vi "HEWH Extract Draw Data.vi"(5 "Test Type":T1, 8 "error in (no error)":errorcluster, 11 "UEF Calculated Values in":T2 {"Data Indexes"."15 sec after Draw Index" format="%#.2f"; "Data Indexes"."15 sec after Draw Timestamp" format="%#.2f"; "Data Indexes"."Test Start Timestamp" format="%.2f"; "Data Indexes"."Test End Timestamp" format="%.2f"; "Data Indexes"."T0 Timestamp" format="%.2f"; "Data Indexes"."Tsf Timestamp" format="%.2f"; "Data Indexes"."Tsu0 Timestamp" format="%.2f"; "Data Indexes"."Tmax1 Timestamp" format="%.2f"; "Data Indexes"."Draw Index Timestamp" format="%#.2f"; "Data Indexes"."Non-Draw Timestamp" format="%#.2f"; "Data Indexes"."Heating Timestamp" format="%#.2f"; "Data Indexes"."Start Energy (BTU-Gas)" format="%.6f"; "Data Indexes"."Start Watt Hours" format="%.6f"; "Static Data"."V - Volume of Wh (True)" format="%.5f"; "Static Data"."T-Ambinet Nominal (°F)" format="%.5f"; "Static Data"."T-Inlet Setpoint (°F)" format="%.5f"; "Static Data"."T-Wh Setpoint (°F)" format="%.5f"; "Sampled Data"."Qe (Wh)" format="%.5f"; "Sampled Data"."Tau stby2 (hr)" format="%.5f"; "Sampled Data"."Tastby2 (°F)" format="%.5f"; "Sampled Data"."Qf (BTU)" format="%.5f"; "Sampled Data"."Qe (BTU)" format="%.5f"; "Sampled Data"."Tmax1 (°F)" format="%.5f"; "Sampled Data"."T0 (°F)" format="%.5f"; "Sampled Data"."Qr (BTU)" format="%.5f"; "Sampled Data"."T 24(°F)" format="%.5f"; "Sampled Data"."T astby(°F)" format="%.5f"; "Sampled Data"."T tstby(°F)" format="%.5f"; "Sampled Data"."T su0(°F)" format="%.5f"; "Sampled Data"."T suf(°F)" format="%.5f"; "Sampled Data"."Tau stby_1 (hr)" format="%.5f"; "Sampled Data"."Qsuf (BTU)" format="%.5f"; "Sampled Data"."Qsu0 (BTU)" format="%.5f"; "Calculated Values"."Draw Bonus Volume (gal)" format="%.6f"; "Calculated Values"."Adjustment Factor" format="%.6f"; "Calculated Values"."T*avg_del(n-1)" format="%.6f"; "Calculated Values"."T*min(n-1)" format="%.6f"; "Calculated Values"."T*avg_del(n)" format="%.6f"; "Calculated Values"."Vn" format="%.6f"; "Calculated Values"."Qdm (BTU)" format="%.6f"; "Calculated Values"."QHWD (BTU)" format="%.6f"; "Calculated Values"."QHW (BTU)" format="%.6f"; "Calculated Values"."UEF" format="%.6f"; "Calculated Values"."QHW67 (BTU)" format="%.6f"; "Calculated Values"."Qda (BTU)" format="%.6f"; "Calculated Values"."Qd (BTU)" format="%.6f"; "Calculated Values"."Q (BTU)" format="%.6f"; "Calculated Values"."UA (BTU/(hr*F))" format="%.6f"; "Calculated Values"."Qhr (BTU/hr)" format="%.6f"; "Calculated Values"."Qstby (BTU)" format="%.6f"; "Calculated Values"."nu_r" format="%.6f"; "Calculated Values"."CpUEF (BTU/(lb*F))" format="%.6f"; "Calculated Values"."rho_nu (lb/gal)" format="%.6f"; "Calculated Values"."V1- Vol (Gal)" format="%.6f"; "Calculated Values"."M cluster mass removed (lb)" format="%.6f"; "Calculated Values"."Cp theoretical (BTU/(lbm °F))" format="%.6f"; "Calculated Values"."Tin1 - Mean Inlet 1st Cluster (°F)" format="%.6f"; "Calculated Values"."Tdel1-Mean Outlet 1st Cluster(°F)" format="%.6f"; "Calculated Values"."Cp 24 (BTU/(lb*F))" format="%.6f"; "Calculated Values"."Cp standby (BTU/(lb*F))" format="%.6f"; "Calculated Values"."Cp2 (BTU/(lb*F))" format="%.6f"; "Calculated Values"."Cp1 (BTU/(lb*F))" format="%.6f"; "Calculated Values"."rho 24 (lb/gal)" format="%.6f"; "Calculated Values"."rho standby (lb/gal)" format="%.6f"; "Calculated Values"."rho 2 (lb/gal)" format="%.6f"; "Calculated Values"."Density of cold water All (lbm/gal)" format="%#.3g"; "Calculated Values"."CpHW (BTU/(lbm °F))" format="%#.3g"; "Calculated Values"."Density of hot water All (lbm/gal)" format="%#.3g"; "Calculated Values"."Mass of water All (lbm)" format="%#.3f"}) -> (0 "error out":errorcluster, 3 "UEF Calculated Values Out":T2 {"Data Indexes"."15 sec after Draw Index" format="%#.2f"; "Data Indexes"."15 sec after Draw Timestamp" format="%#.2f"; "Data Indexes"."Test Start Timestamp" format="%.2f"; "Data Indexes"."Test End Timestamp" format="%.2f"; "Data Indexes"."T0 Timestamp" format="%.2f"; "Data Indexes"."Tsf Timestamp" format="%.2f"; "Data Indexes"."Tsu0 Timestamp" format="%.2f"; "Data Indexes"."Tmax1 Timestamp" format="%.2f"; "Data Indexes"."Draw Index Timestamp" format="%#.2f"; "Data Indexes"."Non-Draw Timestamp" format="%#.2f"; "Data Indexes"."Heating Timestamp" format="%#.2f"; "Data Indexes"."Start Energy (BTU-Gas)" format="%.6f"; "Data Indexes"."Start Watt Hours" format="%.6f"; "Static Data"."V - Volume of Wh (True)" format="%.5f"; "Static Data"."T-Ambinet Nominal (°F)" format="%.5f"; "Static Data"."T-Inlet Setpoint (°F)" format="%.5f"; "Static Data"."T-Wh Setpoint (°F)" format="%.5f"; "Sampled Data"."Qe (Wh)" format="%.5f"; "Sampled Data"."Tau stby2 (hr)" format="%.5f"; "Sampled Data"."Tastby2 (°F)" format="%.5f"; "Sampled Data"."Qf (BTU)" format="%.5f"; "Sampled Data"."Qe (BTU)" format="%.5f"; "Sampled Data"."Tmax1 (°F)" format="%.5f"; "Sampled Data"."T0 (°F)" format="%.5f"; "Sampled Data"."Qr (BTU)" format="%.5f"; "Sampled Data"."T 24(°F)" format="%.5f"; "Sampled Data"."T astby(°F)" format="%.5f"; "Sampled Data"."T tstby(°F)" format="%.5f"; "Sampled Data"."T su0(°F)" format="%.5f"; "Sampled Data"."T suf(°F)" format="%.5f"; "Sampled Data"."Tau stby_1 (hr)" format="%.5f"; "Sampled Data"."Qsuf (BTU)" format="%.5f"; "Sampled Data"."Qsu0 (BTU)" format="%.5f"; "Calculated Values"."Draw Bonus Volume (gal)" format="%.6f"; "Calculated Values"."Adjustment Factor" format="%.6f"; "Calculated Values"."T*avg_del(n-1)" format="%.6f"; "Calculated Values"."T*min(n-1)" format="%.6f"; "Calculated Values"."T*avg_del(n)" format="%.6f"; "Calculated Values"."Vn" format="%.6f"; "Calculated Values"."Qdm (BTU)" format="%.6f"; "Calculated Values"."QHWD (BTU)" format="%.6f"; "Calculated Values"."QHW (BTU)" format="%.6f"; "Calculated Values"."UEF" format="%.6f"; "Calculated Values"."QHW67 (BTU)" format="%.6f"; "Calculated Values"."Qda (BTU)" format="%.6f"; "Calculated Values"."Qd (BTU)" format="%.6f"; "Calculated Values"."Q (BTU)" format="%.6f"; "Calculated Values"."UA (BTU/(hr*F))" format="%.6f"; "Calculated Values"."Qhr (BTU/hr)" format="%.6f"; "Calculated Values"."Qstby (BTU)" format="%.6f"; "Calculated Values"."nu_r" format="%.6f"; "Calculated Values"."CpUEF (BTU/(lb*F))" format="%.6f"; "Calculated Values"."rho_nu (lb/gal)" format="%.6f"; "Calculated Values"."V1- Vol (Gal)" format="%.6f"; "Calculated Values"."M cluster mass removed (lb)" format="%.6f"; "Calculated Values"."Cp theoretical (BTU/(lbm °F))" format="%.6f"; "Calculated Values"."Tin1 - Mean Inlet 1st Cluster (°F)" format="%.6f"; "Calculated Values"."Tdel1-Mean Outlet 1st Cluster(°F)" format="%.6f"; "Calculated Values"."Cp 24 (BTU/(lb*F))" format="%.6f"; "Calculated Values"."Cp standby (BTU/(lb*F))" format="%.6f"; "Calculated Values"."Cp2 (BTU/(lb*F))" format="%.6f"; "Calculated Values"."Cp1 (BTU/(lb*F))" format="%.6f"; "Calculated Values"."rho 24 (lb/gal)" format="%.6f"; "Calculated Values"."rho standby (lb/gal)" format="%.6f"; "Calculated Values"."rho 2 (lb/gal)" format="%.6f"; "Calculated Values"."Density of cold water All (lbm/gal)" format="%#.3g"; "Calculated Values"."CpHW (BTU/(lbm °F))" format="%#.3g"; "Calculated Values"."Density of hot water All (lbm/gal)" format="%#.3g"; "Calculated Values"."Mass of water All (lbm)" format="%#.3f"})   [LabVIEW 2023]
uses:
  Type Definitions/UEF Constants.ctl
  Type Definitions/HEWH Draw Stats.ctl
  Type Definitions/HEWH FHR Draw Type.ctl
  Type Definitions/FHR Bins.ctl
  Type Definitions/HEWH Meter Type.ctl
  Type Definitions/HEWH Test Type.ctl
  Type Definitions/HEWH Remove 15 Seconds.ctl
  <vilib>/Analysis/baseanly.llb/Mean (DBL).vi
  <vilib>/Analysis/NI_AALBase.lvlib
panel:
  # "FHR"
  # "FHR"
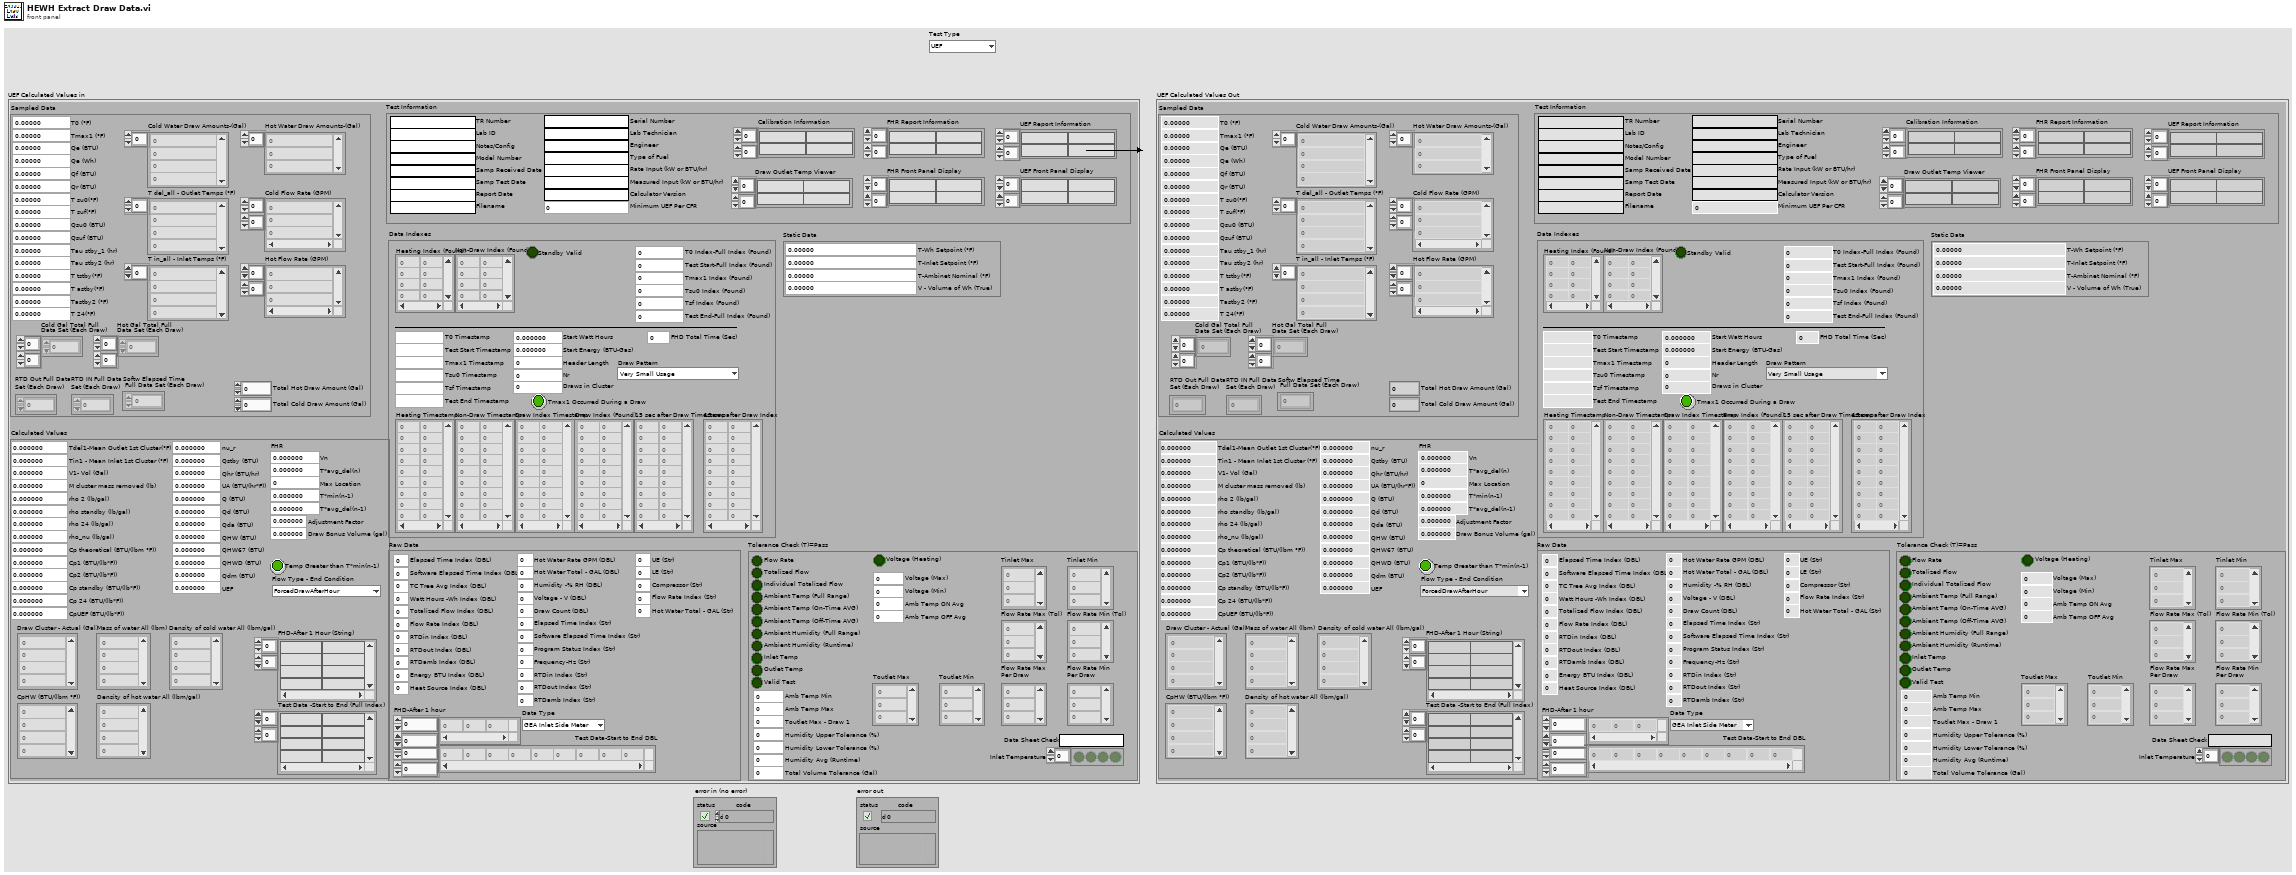
[diagram p1: front panel]
types:
  T1 = typedef "HEWH Test Type.ctl" = enum16{"UEF", "FHD"}
  T2 = typedef "UEF Constants.ctl" = cluster{"Calculated Values":T3, "Sampled Data":cluster{"Cold Water Draw Amounts-(Gal)":dbl[], "T del_all - Outlet Temps (°F)":dbl[], "T in_all - Inlet Temps (°F)":dbl[], "Qsu0 (BTU)":dbl, "Qsuf (BTU)":dbl, "Tau stby_1 (hr)":dbl, "T suf(°F)":dbl, "T su0(°F)":dbl, "T tstby(°F)":dbl, "T astby(°F)":dbl, "T 24(°F)":dbl, "Qr (BTU)":dbl, "T0 (°F)":dbl, "Tmax1 (°F)":dbl, "Qe (BTU)":dbl, "Qf (BTU)":dbl, "Tastby2 (°F)":dbl, "RTD Out Full Data\nSet (Each Draw)":dbl[][], "RTD IN Full Data\nSet (Each Draw)":dbl[][], "Tau stby2 (hr)":dbl, "Hot Water Draw Amounts-(Gal)":dbl[], "Cold Flow Rate (GPM)":dbl[][], "Hot Flow Rate (GPM)":dbl[][], "Softw Elapsed Time\n Full Data Set (Each Draw)":dbl[][], "Cold Gal Total Full\nData Set (Each Draw)":dbl[][], "Total Hot Draw Amount (Gal) ":dbl, "Total Cold Draw Amount (Gal)":dbl, "Qe (Wh)":dbl, "Hot Gal Total Full\nData Set (Each Draw)":dbl[][]}, "Static Data":cluster{"T-Wh Setpoint (°F)":dbl, "T-Inlet Setpoint (°F)":dbl, "T-Ambinet Nominal (°F)":dbl, "V - Volume of Wh (True)":dbl}, "Data Indexes":cluster{"Test Start-Full Index (Found)":i32, "Header Length":i32, "Draw Index (Found)":i32[][], "Nr":i32, "Start Watt Hours":dbl, "Tsu0 Index (Found)":i32, "Tsf Index (Found)":i32, "Start Energy (BTU-Gas)":dbl, "Draws in Cluster":i32, "T0 Index-Full Index (Found)":i32, "Non-Draw Index (Found)":i32[][], "Tmax1 Index (Found)":i32, "Test End-Full Index (Found)":i32, "Heating Index (Found)":i32[][], "Heating Timestamp":dbl[][], "Non-Draw Timestamp":dbl[][], "Draw Index Timestamp":dbl[][], "Tmax1 Timestamp":dbl, "Tsu0 Timestamp":dbl, "Tsf Timestamp":dbl, "T0 Timestamp":dbl, "Test End Timestamp":dbl, "Test Start Timestamp":dbl, "15 sec after Draw Timestamp":dbl[][], "15 sec after Draw Index":dbl[][], "Tmax1 Occurred During a Draw":bool, "FHD Total Time (Sec)":dbl, "Draw Pattern":T5, "Standby Valid":bool}, "Raw Data":cluster{"Elapsed Time Index (DBL)":i32, "Software Elapsed Time Index (DBL)":i32, "TC Tree Avg Index (DBL)":i32, "Watt Hours -Wh Index (DBL)":i32, "Energy BTU Index (DBL)":i32, "Totalized Flow Index (DBL)":i32, "Flow Rate Index (DBL)":i32, "Program Status Index (Str)":i32, "RTDin Index (DBL)":i32, "RTDout Index (DBL)":i32, "RTDamb Index (DBL)":i32, "Test Data-Start to End DBL":dbl[][], "Data Type":T6, "Heat Source Index (DBL)":i32, "Hot Water Rate GPM (DBL)":i32, "Hot Water Total - GAL (DBL)":i32, "FHD-After 1 hour":dbl[][], "Humidity -% RH (DBL)":i32, "Voltage - V (DBL)":i32, "Draw Count (DBL)":i32, "Elapsed Time Index (Str)":i32, "Software Elapsed Time Index (Str)":i32, "Frequency-Hz (Str)":i32, "RTDin Index (Str)":i32, "RTDout Index (Str)":i32, "RTDamb Index (Str)":i32, "UE (Str)":i32, "LE (Str)":i32, "Compressor (Str)":i32, "Flow Rate Index (Str)":i32, "Hot Water Total - GAL (Str)":i32}, "Tolerance Check (T)=Pass":cluster{"Flow Rate":bool, "Totalized Flow":bool, "Ambient Temp (Full Range)":bool, "Ambient Humidity (Full Range)":bool, "Inlet Temp":bool, "Outlet Temp":bool, "Valid Test":bool, "Individual Totalized Flow":bool, "Data Sheet Check":string, "Inlet Temperature":bool[], "Tinlet Max":dbl[], "Tinlet Min":dbl[], "Flow Rate Max (Tol)":dbl[], "Flow Rate Min (Tol)":dbl[], "Amb Temp Max":dbl, "Amb Temp Min":dbl, "Toutlet Max - Draw 1":dbl, "Humidity Upper Tolerance (%)":dbl, "Total Volume Tolerance (Gal)":dbl, "Humidity Lower Tolerance (%)":dbl, "Flow Rate Max\nPer Draw":dbl[], "Flow Rate Min\nPer Draw":dbl[], "Ambient Humidity (Runtime)":bool, "Humidity Avg (Runtime)":dbl, "Ambient Temp (On-Time AVG)":bool, "Ambient Temp (Off-Time AVG)":bool, "Amb Temp OFF Avg":dbl, "Amb Temp ON Avg":dbl, "Voltage (Heating)":bool, "Voltage (Min)":dbl, "Voltage (Max)":dbl, "Toutlet Max":dbl[], "Toutlet Min":dbl[]}, "Test Information":cluster{"TR Number":string, "Lab ID":string, "Notes/Config":string, "Model Number":string, "Serial Number":string, "Lab Technician":string, "Engineer":string, "Type of Fuel":string, "Samp Received Date":string, "Samp Test Date":string, "Report Date":string, "Rate Input (kW or BTU/hr)":string, "Measured Input (kW or BTU/hr)":string, "Filename":string, "Calibration Information":string[][], "Calculator Version":string, "Minimum UEF Per CFR":dbl, "UEF Report Information":string[][], "FHR Report Information":string[][], "FHR Front Panel Display":string[][], "UEF Front Panel Display":string[][], "Draw Outlet Temp Viewer":string[][]}}
  T3 = typedef "HEWH Draw Stats.ctl" = cluster{"Draw Cluster - Actual (Gal)":dbl[], "Mass of water All (lbm)":dbl[], "Density of hot water All (lbm/gal)":dbl[], "CpHW (BTU/(lbm °F))":dbl[], "rho 2 (lb/gal)":dbl, "rho standby (lb/gal)":dbl, "rho 24 (lb/gal)":dbl, "Cp1 (BTU/(lb*F))":dbl, "Cp2 (BTU/(lb*F))":dbl, "Cp standby (BTU/(lb*F))":dbl, "Cp 24 (BTU/(lb*F))":dbl, "nu_r":dbl, "Qstby (BTU)":dbl, "Qhr (BTU/hr)":dbl, "UA (BTU/(hr*F))":dbl, "Q (BTU)":dbl, "Qd (BTU)":dbl, "Qda (BTU)":dbl, "QHW67 (BTU)":dbl, "UEF":dbl, "Tdel1-Mean Outlet 1st Cluster(°F)":dbl, "Tin1 - Mean Inlet 1st Cluster (°F)":dbl, "Cp theoretical (BTU/(lbm °F))":dbl, "M cluster mass removed (lb)":dbl, "V1- Vol (Gal)":dbl, "Test Data -Start to End (Full Index)":string[][], "rho_nu (lb/gal)":dbl, "Density of cold water All (lbm/gal)":dbl[], "CpUEF (BTU/(lb*F))":dbl, "QHW (BTU)":dbl, "QHWD (BTU)":dbl, "Qdm (BTU)":dbl, "FHD-After 1 Hour (String)":string[][], "Vn":dbl, "T*avg_del(n)":dbl, "Max Location":i32, "T*min(n-1)":dbl, "T*avg_del(n-1)":dbl, "Temp Greater than T*min(n-1)":bool, "Adjustment Factor":dbl, "Draw Bonus Volume (gal)":dbl, "Flow Type - End Condition":T4}
  T4 = typedef "HEWH FHR Draw Type.ctl" = enum16{"ForcedDrawAfterHour", "HeatingCutoffBeforeHour"}
  T5 = typedef "FHR Bins.ctl" = enum16{"Very Small Usage", "Low Usage", "Medium Usage", "High Usage", "Undefined"}
  T6 = typedef "HEWH Meter Type.ctl" = enum16{"GEA Inlet Side Meter", "GEA Outlet Side Meter", "CSA Inlet Side Meter"}
  T7 = typedef "HEWH Remove 15 Seconds.ctl" = cluster{"Cold Water Total (Gal)":dbl[], "Software Elapsed Time (s)":dbl[], "RTDin (Input)":dbl[], "RTDout (Input)":dbl[], "Cold Flow Rate (GPM)":dbl[], "Hot Flow Rate (GPM)":dbl[], "Hot Water Total (Gal)":dbl[], "Cold Water Draw Amount (Gal)":dbl, "Hot Water Draw Amount (Gal)":dbl, "Draw Index":i32[], "Test Data-Start to End DBL":dbl[][], "Hot Water Total (gal)-Index":i32, "Totalized Flow Index-Index":i32}
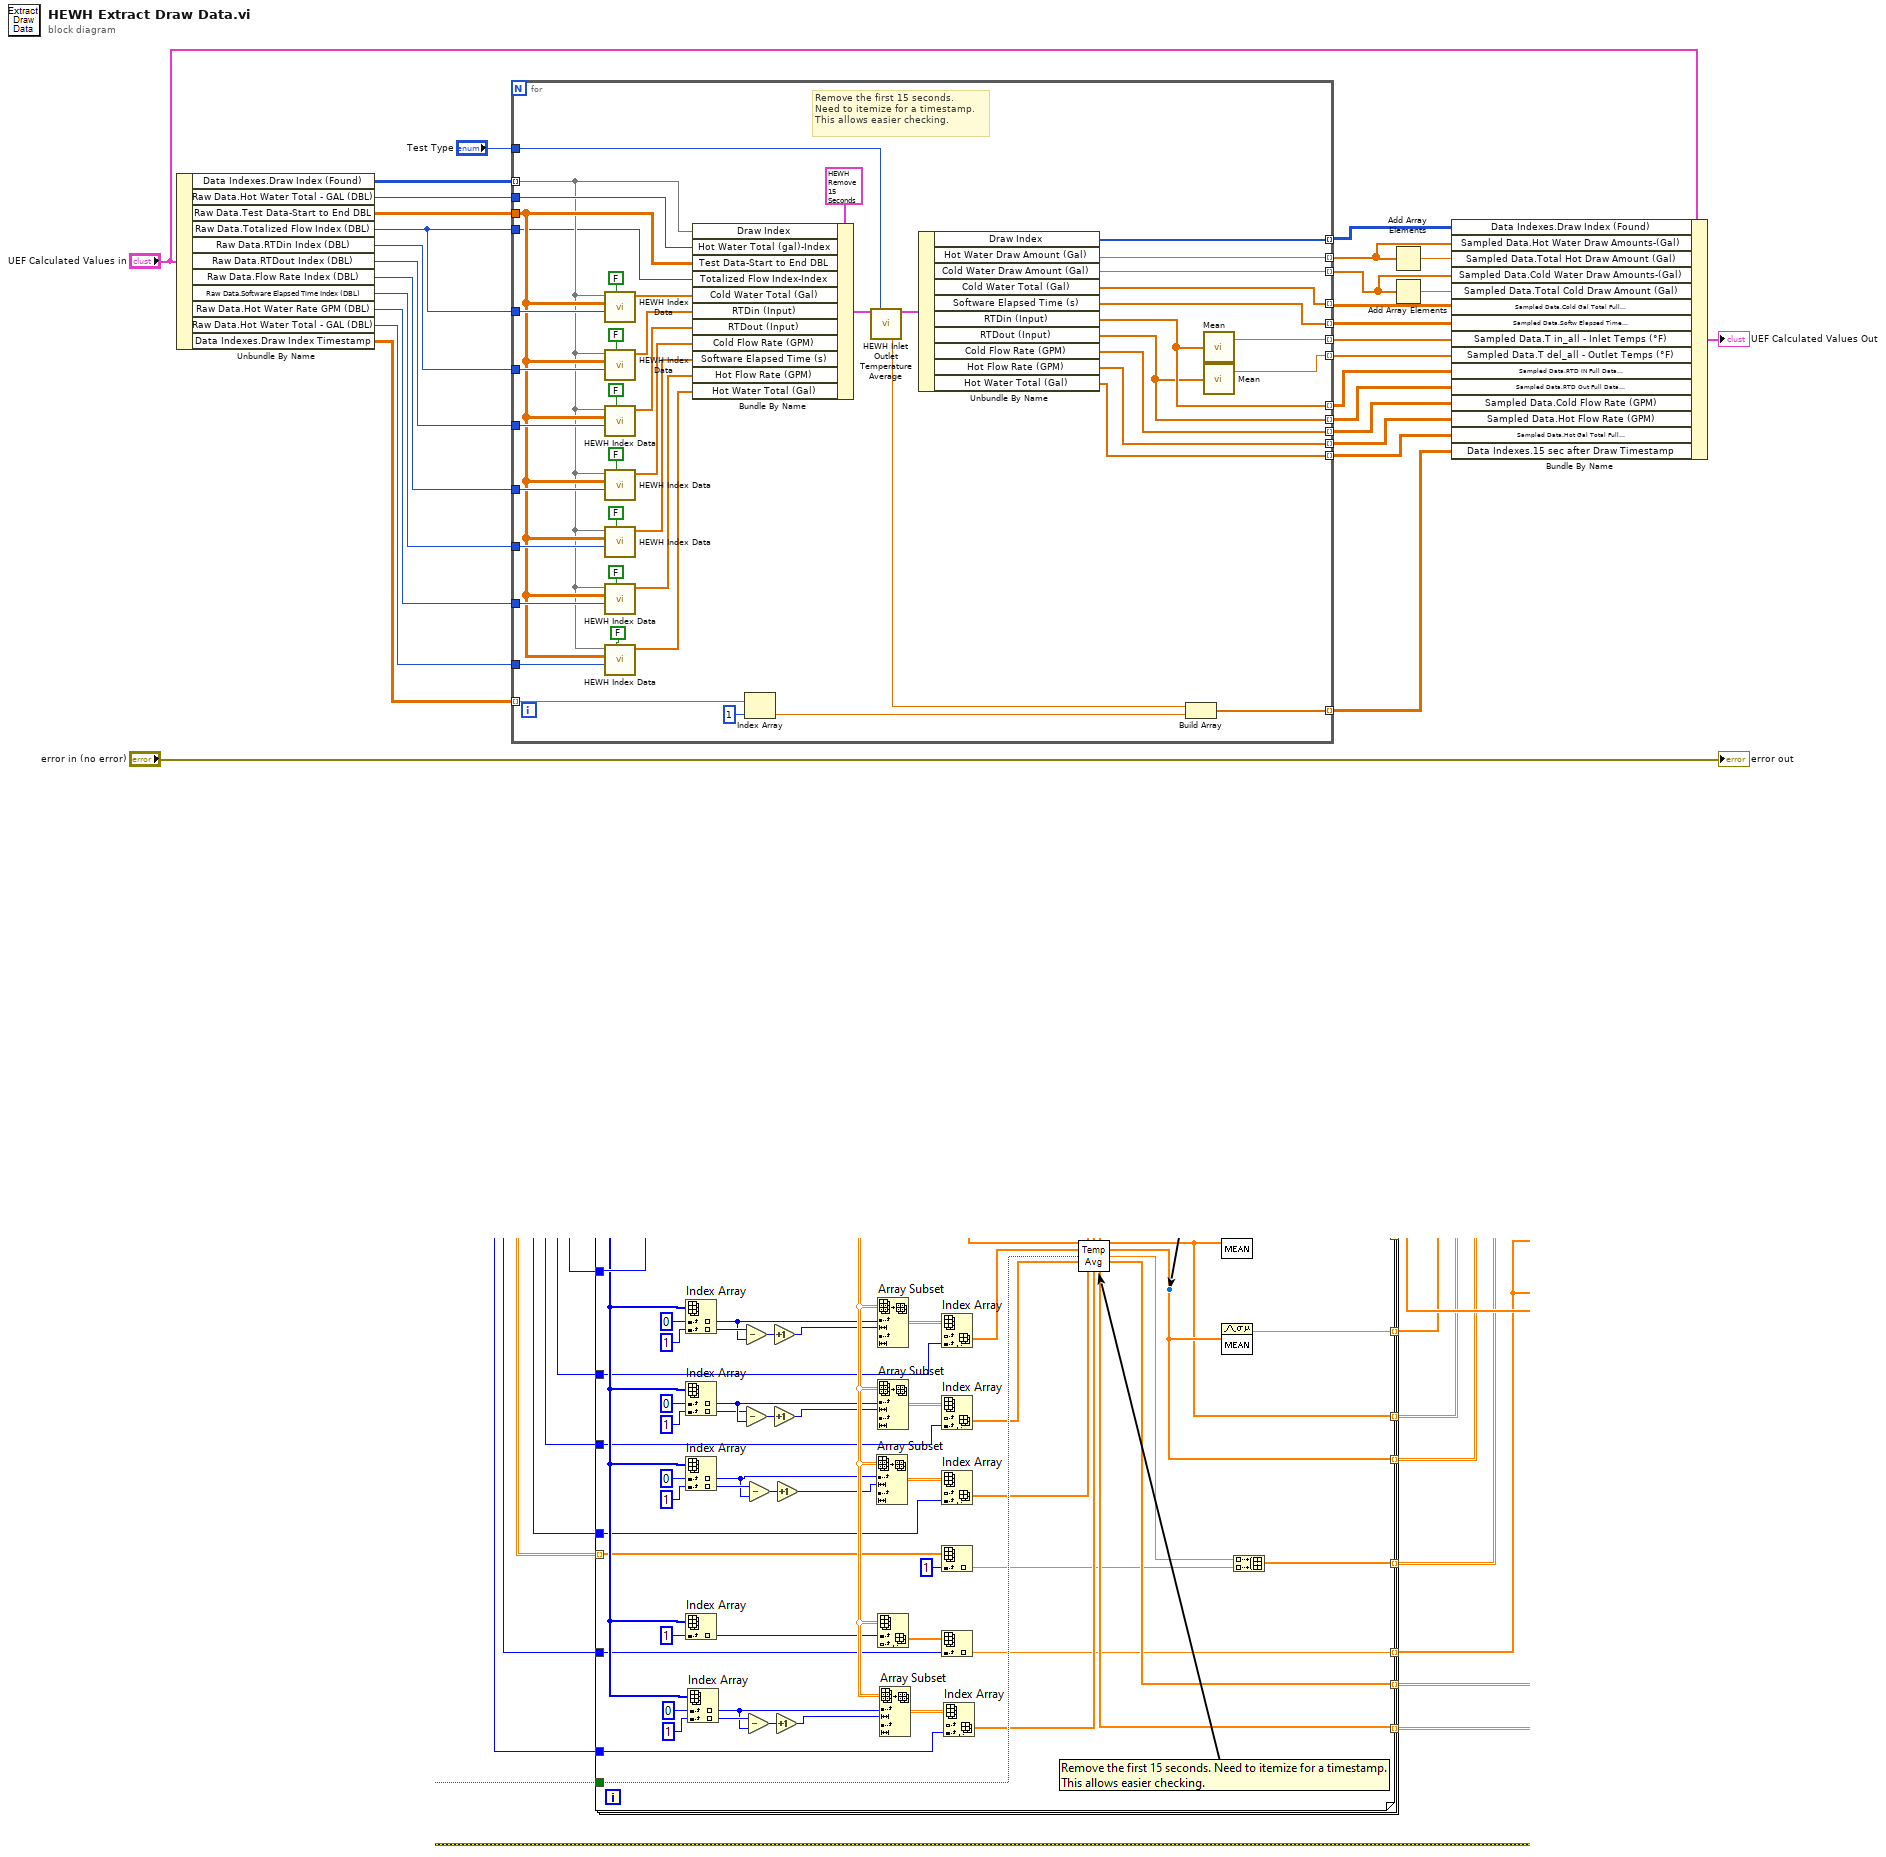
[diagram p0: block diagram]
diagram:
  n1 = Unbundle By Name("UEF Calculated Values in") -> ("Data Indexes.Draw Index (Found)"=w3:i32[][], "Raw Data.Hot Water Total - GAL (DBL)"=w17:i32, "Raw Data.Test Data-Start to End DBL"=w14:dbl[][], "Raw Data.Totalized Flow Index (DBL)"=w16:i32, "Raw Data.RTDin Index (DBL)"=w26:i32, "Raw Data.RTDout Index (DBL)"=w25:i32, "Raw Data.Flow Rate Index (DBL)"=w24:i32, "Raw Data.Software Elapsed Time Index (DBL)"=w23:i32, "Raw Data.Hot Water Rate GPM (DBL)"=w15:i32, "Raw Data.Hot Water Total - GAL (DBL)"=w9:i32, "Data Indexes.Draw Index Timestamp"=w8:dbl[][])
  n2 = for {
    tunnel: w3 -> [w35] mode=indexing
    tunnel: w14 -> [w39]
    tunnel: [w36] -> w11 mode=indexing
    tunnel: [w76] -> w29 mode=indexing
    tunnel: [w75] -> w28 mode=indexing
    tunnel: [w48] -> w18 mode=indexing
    tunnel: [w47] -> w27 mode=indexing
    tunnel: w16 -> [w65]
    tunnel: w26 -> [w70]
    tunnel: w25 -> [w69]
    tunnel: w24 -> [w68]
    tunnel: w23 -> [w67]
    tunnel: w8 -> [w74] mode=indexing
    tunnel: [w72] -> w1 mode=indexing
    tunnel: w17 -> [w38]
    tunnel: [w37] -> w13 mode=indexing
    tunnel: w15 -> [w66]
    tunnel: [w46] -> w22 mode=indexing
    tunnel: [w45] -> w21 mode=indexing
    tunnel: [w49] -> w20 mode=indexing
    tunnel: [w50] -> w19 mode=indexing
    tunnel: w16 -> [w34]
    tunnel: w9 -> [w41]
    tunnel: "Test Type" -> [w33]
    tunnel: [w32] -> w4 mode=indexing
    tunnel: [w31] -> w2 mode=indexing
    # "Remove the first 15 seconds.\nNeed to itemize for a timestamp.\nThis allows easier checking."
    n3 = call "HEWH Index Data.vi"("Basic Index?"=FALSE, "Data Index Location"=w65, "Test Data-Start to End DBL"=w39, "Draw Index"=w35) -> ("Extracted Data"=w57:dbl[])  [unwired: 5 in, 2 out]
    n4 = call "HEWH Index Data.vi"("Basic Index?"=FALSE, "Data Index Location"=w70, "Test Data-Start to End DBL"=w39, "Draw Index"=w35) -> ("Extracted Data"=w56:dbl[])  [unwired: 5 in, 2 out]
    n5 = call "HEWH Index Data.vi"("Basic Index?"=FALSE, "Data Index Location"=w69, "Test Data-Start to End DBL"=w39, "Draw Index"=w35) -> ("Extracted Data"=w55:dbl[])  [unwired: 5 in, 2 out]
    n6 = call "HEWH Index Data.vi"("Basic Index?"=FALSE, "Data Index Location"=w68, "Test Data-Start to End DBL"=w39, "Draw Index"=w35) -> ("Extracted Data"=w54:dbl[])  [unwired: 5 in, 2 out]
    n7 = call "HEWH Index Data.vi"("Basic Index?"=FALSE, "Data Index Location"=w67, "Test Data-Start to End DBL"=w39, "Draw Index"=w35) -> ("Extracted Data"=w53:dbl[])  [unwired: 5 in, 2 out]
    n8 = call "HEWH Index Data.vi"("Basic Index?"=FALSE, "Data Index Location"=w66, "Test Data-Start to End DBL"=w39, "Draw Index"=w35) -> ("Extracted Data"=w52:dbl[])  [unwired: 5 in, 2 out]
    n9 = call "HEWH Index Data.vi"("Basic Index?"=FALSE, "Data Index Location"=w41, "Test Data-Start to End DBL"=w39, "Draw Index"=w35) -> ("Extracted Data"=w40:dbl[])  [unwired: 5 in, 2 out]
    n10 = Bundle By Name(cluster=T7 {"Cold Water Total (Gal)"=[], "Software Elapsed Time (s)"=[], "RTDin (Input)"=[], "RTDout (Input)"=[], "Cold Flow Rate (GPM)"=[], "Hot Flow Rate (GPM)"=[], "Hot Water Total (Gal)"=[], "Cold Water Draw Amount (Gal)"=0.0, "Hot Water Draw Amount (Gal)"=0.0, "Draw Index"=[], "Test Data-Start to End DBL"=[], "Hot Water Total (gal)-Index"=0, "Totalized Flow Index-Index"=0} ("Remove 15 Seconds Input"), "Draw Index"=w35, "Hot Water Total (gal)-Index"=w38, "Test Data-Start to End DBL"=w39, "Totalized Flow Index-Index"=w34, "Cold Water Total (Gal)"=w57, "RTDin (Input)"=w56, "RTDout (Input)"=w55, "Cold Flow Rate (GPM)"=w54, "Software Elapsed Time (s)"=w53, "Hot Flow Rate (GPM)"=w52, "Hot Water Total (Gal)"=w40) -> (w51:T7)
    n11 = Index Array "Index Array"(array=w74, index=1) -> (element=w73:dbl)
    n12 = call "HEWH Inlet Outlet Temperature Average.vi"("Remove 15 Seconds Input"=w51, "Test Type"=w33) -> ("Remove 15 Seconds Output"=w43:T7, "Time_15s"=w44:dbl)  [unwired: 11 in, 1 out]
    n13 = Unbundle By Name(w43) -> ("Draw Index"=w32:i32[], "Hot Water Draw Amount (Gal)"=w37:dbl, "Cold Water Draw Amount (Gal)"=w36:dbl, "Cold Water Total (Gal)"=w50:dbl[], "Software Elapsed Time (s)"=w49:dbl[], "RTDin (Input)"=w48:dbl[], "RTDout (Input)"=w47:dbl[], "Cold Flow Rate (GPM)"=w46:dbl[], "Hot Flow Rate (GPM)"=w45:dbl[], "Hot Water Total (Gal)"=w31:dbl[])
    n14 = Build Array(w44, w73) -> (w72:dbl[])
    n15 = call-poly <vilib>:"Mean.vi"("X"=w48) -> ("mean"=w76:dbl)  [unwired: 1 out]
    n16 = call-poly <vilib>:"Mean.vi"("X"=w47) -> ("mean"=w75:dbl)  [unwired: 1 out]
  }
  n17 = Add Array Elements(numeric array=w13) -> (sum=w12:dbl)
  n18 = Add Array Elements(numeric array=w11) -> (sum=w10:dbl)
  n19 = Bundle By Name(cluster="UEF Calculated Values in", "Data Indexes.Draw Index (Found)"=w4, "Sampled Data.Hot Water Draw Amounts-(Gal)"=w13, "Sampled Data.Total Hot Draw Amount (Gal)"=w12, "Sampled Data.Cold Water Draw Amounts-(Gal)"=w11, "Sampled Data.Total Cold Draw Amount (Gal)"=w10, "Sampled Data.Cold Gal Total Full\nData Set (Each Draw)"=w19, "Sampled Data.Softw Elapsed Time\n Full Data Set (Each Draw)"=w20, "Sampled Data.T in_all - Inlet Temps (°F)"=w29, "Sampled Data.T del_all - Outlet Temps (°F)"=w28, "Sampled Data.RTD IN Full Data\nSet (Each Draw)"=w18, "Sampled Data.RTD Out Full Data\nSet (Each Draw)"=w27, "Sampled Data.Cold Flow Rate (GPM)"=w22, "Sampled Data.Hot Flow Rate (GPM)"=w21, "Sampled Data.Hot Gal Total Full\nData Set (Each Draw)"=w2, "Data Indexes.15 sec after Draw Timestamp"=w1) -> (→"UEF Calculated Values Out":T2)
  "error out" <- "error in (no error)"
